vi "pause.vi"(0 "Dataflow In":errorcluster, 1 "Pause":refnum<vi>) -> (5 "Dataflow Out":errorcluster)   [LabVIEW 2019]
uses:
  lib/libSimulationControl/libSimulationControl.lvlib
panel:
  # "*******************************************************************\nBiogas Plant Control\n\nAuthor: Paul Zügel\nGCSC-Frankfurt am Main 2020\n\n*******************************************************************"
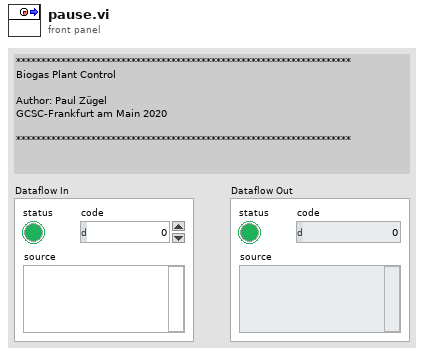
[diagram p1: front panel]
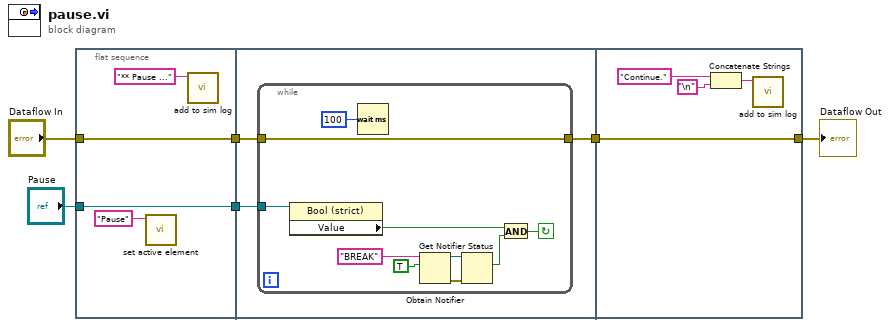
[diagram p0: block diagram]
diagram:
  n1 = flat-sequence {
    tunnel: "Pause" -> [w9]
    tunnel: "Dataflow In" -> [w10]
    tunnel: [w10] -> w5
    tunnel: [w9] -> w4
    tunnel: w5 -> [w13]
    tunnel: w4 -> [w11]
    tunnel: [w12] -> w3
    tunnel: [w27] -> w1
    tunnel: w3 -> [w27]
    frame #0 {
      n2 = call "set active element.vi"("elem"="Pause") -> ()  [unwired: 10 in, 1 out]
      n3 = call "add to sim log.vi"("log"="** Pause ..." ("string")) -> ()  [unwired: 10 in, 1 out]
    }
    frame #1 {
      n4 = while {
        tunnel: w13 -> [w22]
        tunnel: [w22] -> w12
        tunnel: w11 -> [w21]
        stop <- w14 continue-if-true
        n5 = property class="Bool (strict)"(reference=w21) -> ("Value"=w16:bool)  [unwired: 1 in, 2 out]
        n6 = Wait (ms)(milliseconds to wait=u32 100) -> ()  [unwired: 1 out]
        n7 = Obtain Notifier(name (unnamed)="BREAK", notification data type=TRUE) -> (notifier out=w18:refnum<notifier>, error out=w17:errorcluster)  [unwired: 2 in, 1 out]
        n8 = Get Notifier Status(notifier=w18, error in (no error)=w17) -> (current notification=w15:bool)  [unwired: 4 out]
        n9 = And(x=w16, y=w15) -> (x .and. y?=w14:bool)
      }
    }
    frame #2 {
      n10 = Concatenate Strings("Continue." ("string"), "\n") -> (w24:string)
      n11 = call "add to sim log.vi"("log"=w24) -> ()  [unwired: 10 in, 1 out]
    }
  }
  "Dataflow Out" <- w1
